vi "Write Application.vi"(8 "error in (no error)":errorcluster, 10 "Application":refnum<k7>, 11 "Asylum_Driver in":refnum<class "Asylum_Driver.lvclass">) -> (0 "error out":errorcluster, 3 "Asylum_Driver out":refnum<class "Asylum_Driver.lvclass">)   [LabVIEW 2019, in "Asylum_Driver.lvclass"]
uses:
  Asylum_Driver.lvclass
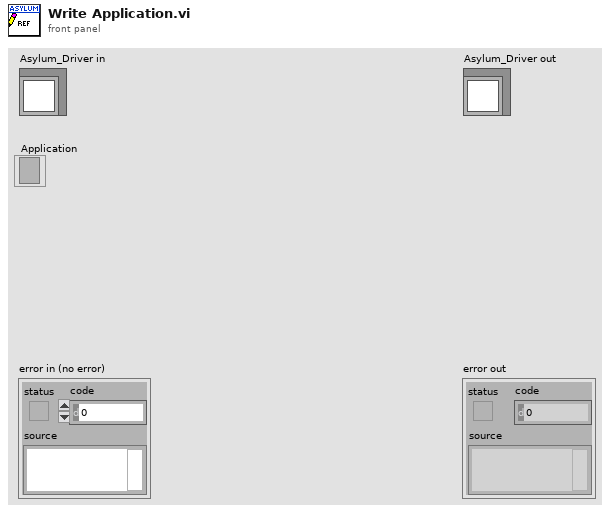
[diagram p1: front panel]
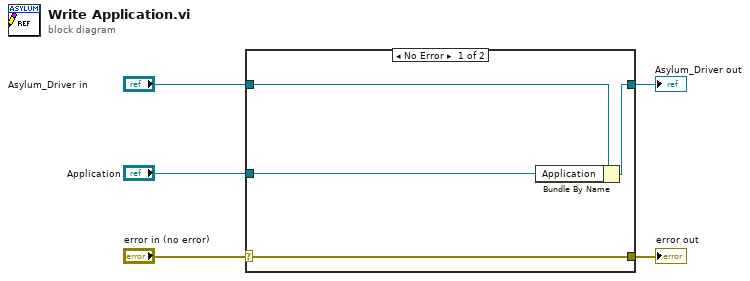
[diagram p0: block diagram]
diagram:
  n1 = case shown="No Error" "error in (no error)" {
    selector: "error in (no error)" -> [w9 w10]
    tunnel: [w9 w10] -> w4
    tunnel: [w7 w11] -> w2
    tunnel: "Asylum_Driver in" -> [w8 w11]
    tunnel: "Application" -> [w6 _]
    frame No Error {
      n2 = Bundle By Name(cluster=w8, "Application"=w6) -> (w7:refnum<class "Asylum_Driver.lvclass">)
    }
    frame Error {
    }
  }
  "error out" <- w4
  "Asylum_Driver out" <- w2
